vi "DWordToHex.vi"(11 "DWORD":i32[](array[numeric])) -> (3 "数组":u16[](array[numeric]) format="%04xH")   [LabVIEW 2016, in "氨氮.lvlib"]
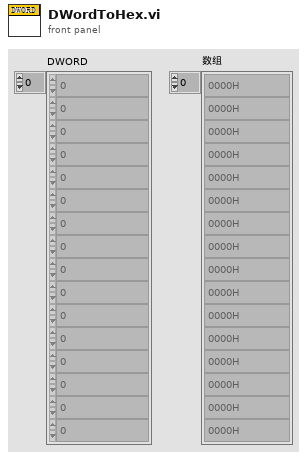
[diagram p1: front panel]
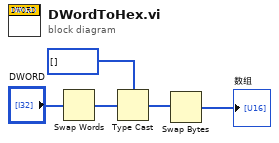
[diagram p0: block diagram]
diagram:
  n1 = Swap Words(1:"DWORD") -> (0:w4:i32[])
  n2 = Type Cast(type=u16[] [] ("数组"), x=w4) -> (*(type *) &x=w2:u16[])
  n3 = Swap Bytes(anything=w2) -> (byte swapped=→"数组":u16[])
